vi "Single Write.vi"(7 "Data":i32, 8 "error in (no error)":errorcluster, 10 "Start Register":i32, 11 "Slave Address":i32) -> (0 "error out":errorcluster, 2 "Command":string)   [LabVIEW 2014, in "Modbus.lvlib"]
uses:
  Modbus.lvlib
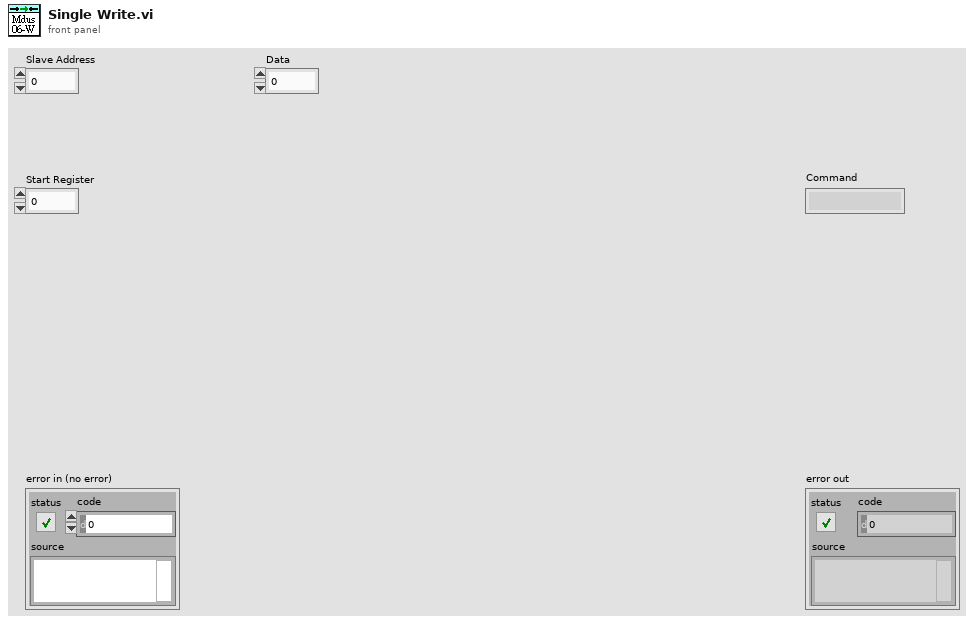
[diagram p1: front panel]
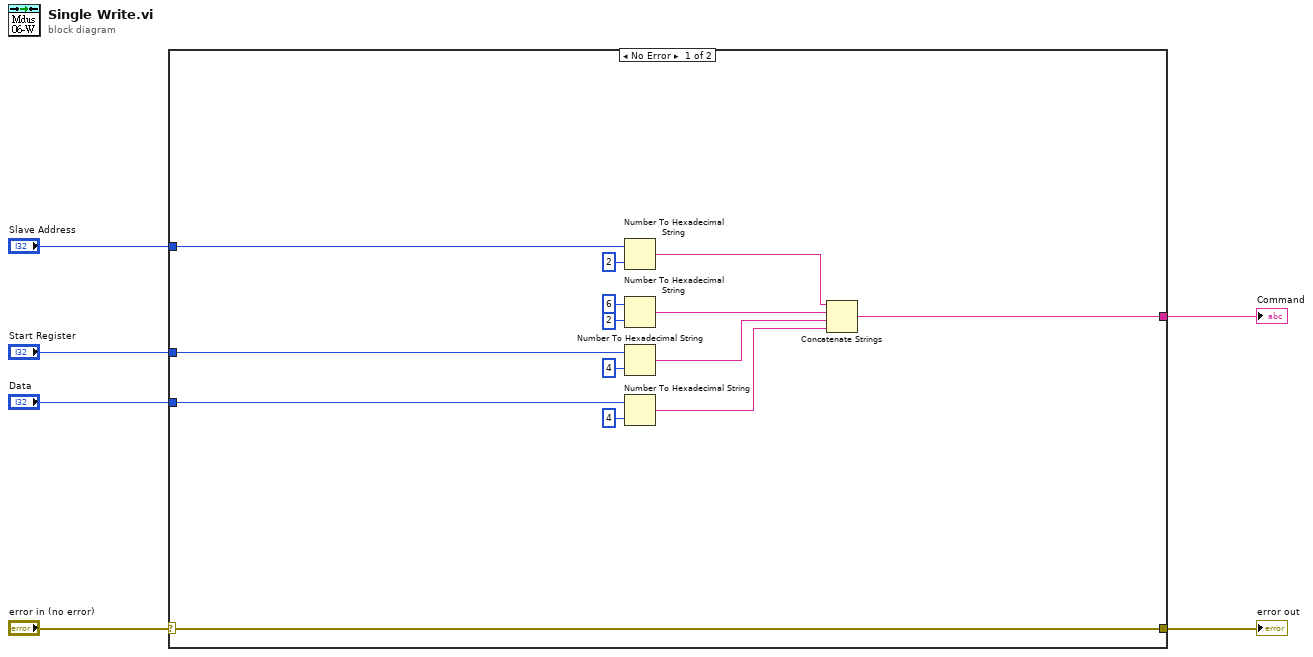
[diagram p0: block diagram]
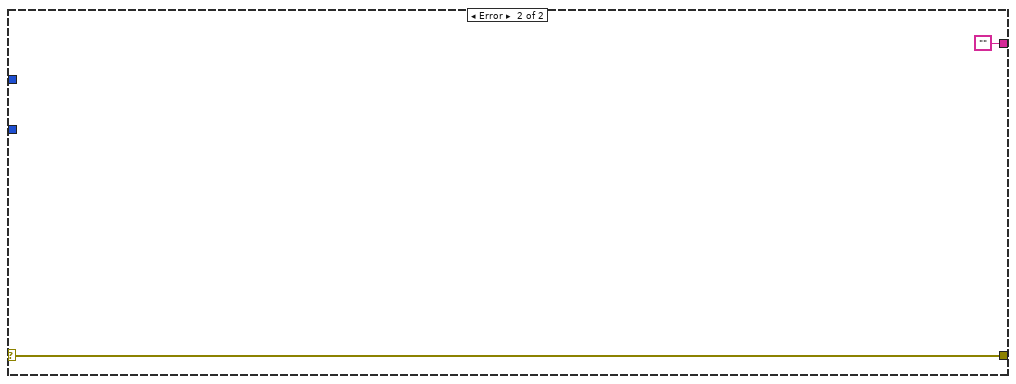
[diagram p2: hidden frame]
diagram:
  n1 = case shown="No Error" "error in (no error)" {
    selector: "error in (no error)" -> [w20 w22]
    tunnel: [w20 w22] -> w5
    tunnel: "Slave Address" -> [w10 _]
    tunnel: "Start Register" -> [w9 _]
    tunnel: "Data" -> [w8 _]
    tunnel: [w7 ""] -> w1
    frame No Error {
      n2 = Number To Hexadecimal String(1:i16 2 ("width (-)"), 2:w10) -> (0:w15:string)
      n3 = Number To Hexadecimal String(1:i16 2 ("width (-)"), 2:6 ("number")) -> (0:w14:string)
      n4 = Number To Hexadecimal String(1:i16 4 ("width (-)"), 2:w9) -> (0:w13:string)
      n5 = Number To Hexadecimal String(1:i16 4 ("width (-)"), 2:w8) -> (0:w11:string)
      n6 = Concatenate Strings(w15, w14, w13, w11) -> (w7:string)
    }
    frame Error {
    }
  }
  "error out" <- w5
  "Command" <- w1
